vi "sine Pattern vs Sine Waveform.vi"() -> ()   [LabVIEW 2020]
uses:
  <vilib>/measure/NI_MABase.lvlib
  <vilib>/Analysis/NI_AALBase.lvlib
panel:
  out "1/x":dbl
  in  "Fs":dbl
  in  "samples":i32=128
  in  "cycles":dbl=1.0 format="%0.2f"
  out "Sine Pattern":waveform(dbl)(graph)
  in  "phase":dbl format="%.2p"
  out "Sine Waveform":waveform(dbl)(graph)
  in  "frequency":dbl=10.0 format="%0.2p"
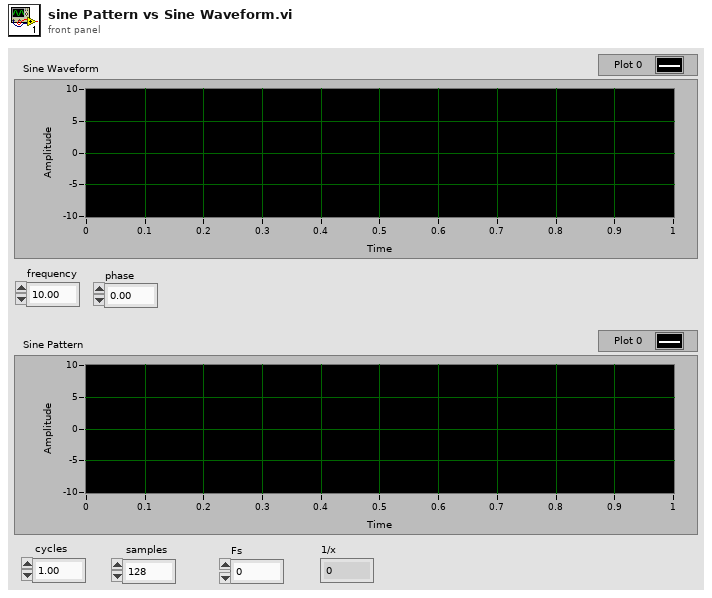
[diagram p1: front panel]
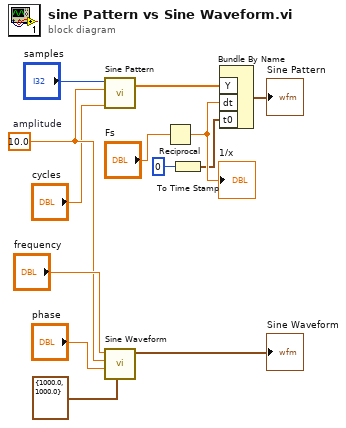
[diagram p0: block diagram]
diagram:
  w10 = 10.0  # amplitude
  n1 = call <vilib>:"Sine Pattern.vi"("cycles"="cycles", "amplitude"=w10, "samples"="samples") -> ("Sinusoidal Pattern"=w6:dbl[])  [unwired: 1 in, 1 out]
  n2 = call <vilib>:"Sine Waveform.vi"("sampling info"=cluster{"Fs":dbl, "#s":dbl} {"Fs"=1000.0, "#s"=1000.0}, "phase"="phase", "amplitude"=w10, "frequency"="frequency") -> ("signal out"=→"Sine Waveform":waveform(dbl))  [unwired: 6 in, 1 out]
  n3 = Reciprocal(x="Fs") -> (1/x=w3:dbl)
  "1/x" <- w3
  n4 = To Time Stamp(1:0) -> (0:w1:timestamp)
  n5 = Bundle By Name("Y"=w6, "dt"=w3, "t0"=w1) -> (→"Sine Pattern":waveform(dbl))  [unwired: 1 in]
